vi "Get TimeStamp from NTP.vi"(8 "error in (no error)":errorcluster, 11 "Time Server\nIP Address":string="192.168.1.43") -> (0 "error out":errorcluster, 1 "Time Server\nUsed":string, 2 "Time Server\nRequested":string, 3 "Returned\nTime Stamp":timestamp format="%<%c>T")   [LabVIEW 2011]
doc: "Gets the time using the NTP protocol and sets the RT clock to that time"
uses:
  <vilib>/NI_Real-Time Target Support.lvlib
panel:
  in  "Inhibit inverse DNS":bool=TRUE
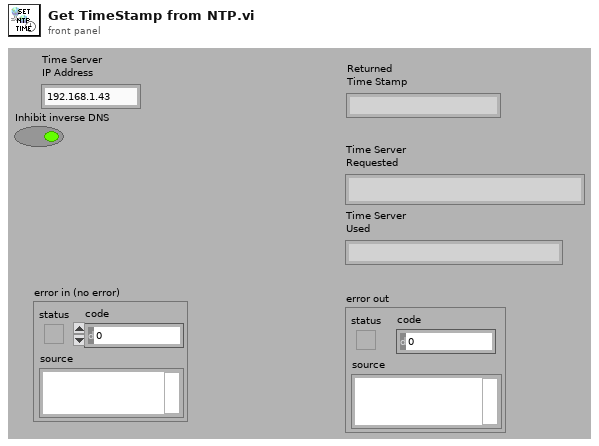
[diagram p1: front panel]
types:
  T1 = typedef "LVDateTimeRec.ctl" = cluster{"fractional second":dbl, "second":i32, "minute":i32, "hour":i32, "day of month":i32, "month":i32, "year":i32, "day of week":i32, "day of year":i32, "DST":i32}
  T2 = enum16{"set date", "set local time", "set UTC time"}
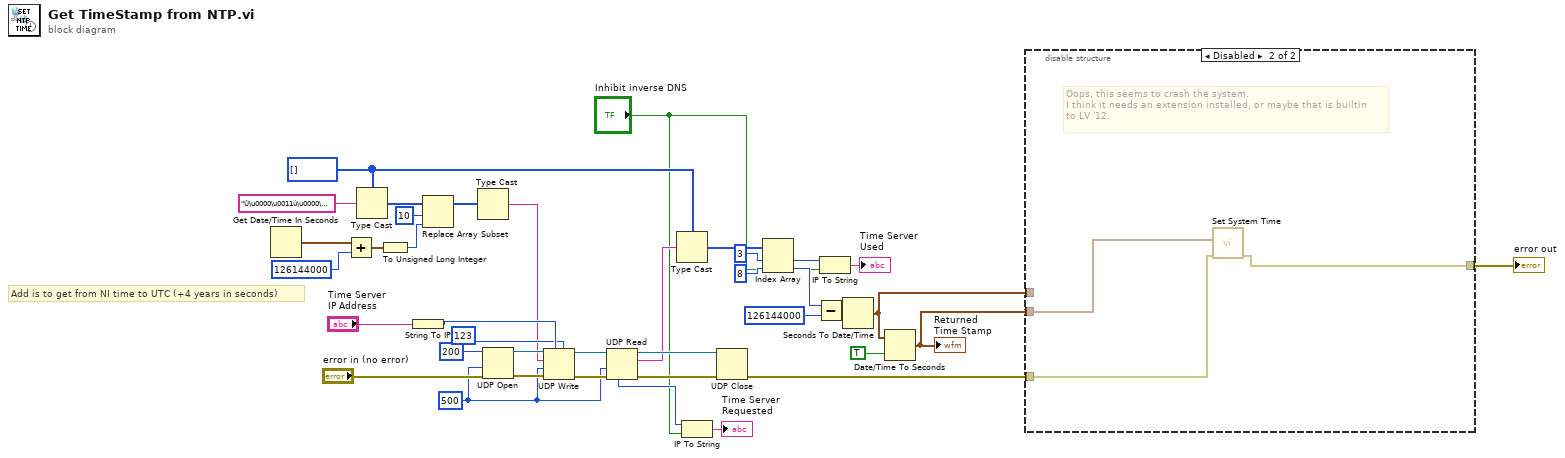
[diagram p0: block diagram]
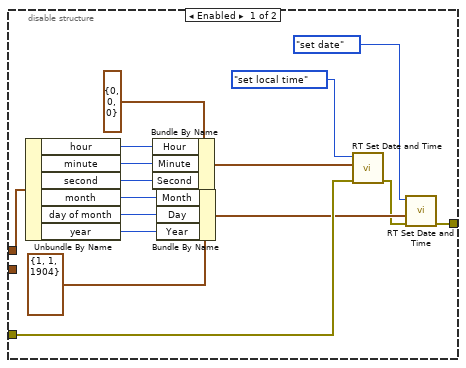
[diagram p2: hidden frame]
diagram:
  w3 = 500 ("timeout ms (25000)")
  w6 = u32[] []
  # "Add is to get from NI time to UTC (+4 years in seconds)"
  n1 = Get Date/Time In Seconds() -> (seconds since 1Jan1904=w24:timestamp)
  n2 = Add(x=w24, y=u32 126144000) -> (x+y=w19:timestamp)
  n3 = Type Cast(type=w6, x="Û\u0000\u0011ú\u0000\u0000\u0000\u0000\u0000\u0001\u0003þ\u0000\u0000\u0000\u0000Ð!ú*\u0017KÆ§\u0000\u0000\u0000\u0000\u0000\u0000\u0000\u0000\u0000\u0000\u0000\u0000\u0000\u0000\u0000\u0000Ð'l\u001a‚MÒñ€:\u0000\u0000\u0000\u0000\u0000\u0000\u0000\u0000\u0000\u0000\u0000\u0000\u0000\u0000\u0000\u0000\u0000\u0000" ("String")) -> (*(type *) &x=w22:u32[])
  n4 = To Unsigned Long Integer(number=w19) -> (unsigned 32bit integer=w13:u32)
  n5 = String To IP(1:"Time Server\nIP Address") -> (0:w36:u32)
  n6 = Replace Array Subset(array=w22, new element=w13, index=10) -> (w21:u32[])
  n7 = Type Cast(x=w21) -> (*(type *) &x=w16:string)  [unwired: 1 in]
  n8 = UDP Open(8:"error in (no error)", 9:w3, 11:u16 200 ("port")) -> (port=w37:refnum<k16>, 0:w38:errorcluster)  [unwired: 2 in, 1 out]
  n9 = UDP Write(address=w36, port or service name=u16 123 ("port"), connection ID=w37, data in=w16, 8:w38, 9:w3) -> (error out=w35:errorcluster, 3:w34:refnum<k16>)
  n10 = UDP Read(connection ID=w34, timeout ms (25000)=w3, 8:w35) -> (data out=w27:string, error out=w32:errorcluster, 3:w33:refnum<k16>, 6:w29:u32)  [unwired: 1 in, 1 out]
  n11 = Type Cast(type=w6, x=w27) -> (*(type *) &x=w26:u32[])
  n12 = IP To String(1:"Inhibit inverse DNS", 2:w29) -> (0:→"Time Server\nRequested":string)
  n13 = UDP Close(connection ID=w33, 8:w32) -> (error out=w11:errorcluster)  [unwired: 1 out]
  n14 = Index Array(array=w26, index #1=3 ("index"), index #2=8 ("index")) -> (element #1=w12:u32, element #2=w8:u32)
  n15 = Subtract(x=w8, y=u32 126144000) -> (x-y=w15:u32)
  n16 = IP To String(1:"Inhibit inverse DNS", 2:w12) -> (0:→"Time Server\nUsed":string)
  n17 = Seconds To Date/Time(time stamp (now)=w15) -> (date time rec=w5:T1)  [unwired: 1 in]
  n18 = Date/Time To Seconds(1:TRUE ("is UTC (F)"), 2:w5) -> (0:w1:timestamp)
  "Returned\nTime Stamp" <- w1
  n19 = disable-structure shown="Disabled" {
    disable-tunnel: w11 -> [w50 w58]
    disable-tunnel: [w44 w57] -> w10
    disable-tunnel: w5 -> [w43 _]
    disable-tunnel: w1 -> [_ w56]
    frame Enabled {
      n20 = Unbundle By Name(w43) -> ("hour"=w53:i32, "minute"=w52:i32, "second"=w51:i32, "month"=w48:i32, "day of month"=w47:i32, "year"=w46:i32)
      n21 = Bundle By Name(cluster=cluster{"Hour":i32, "Minute":i32, "Second":i32} {"Hour"=0, "Minute"=0, "Second"=0} ("Time"), "Hour"=w53, "Minute"=w52, "Second"=w51) -> (w54:cluster{"Hour":i32, "Minute":i32, "Second":i32})
      n22 = Bundle By Name(cluster=cluster{"Month":i32, "Day":i32, "Year":i32} {"Month"=1, "Day"=1, "Year"=1904} ("Date"), "Month"=w48, "Day"=w47, "Year"=w46) -> (w45:cluster{"Month":i32, "Day":i32, "Year":i32})
      n23 = call <vilib>:"RT Set Date and Time.vi"("error in (no error)"=w50, "Time"=w54, "mode"=T2."set local time") -> ("error out"=w41:errorcluster)  [unwired: 8 in]
      n24 = call <vilib>:"RT Set Date and Time.vi"("error in (no error)"=w41, "Date"=w45, "mode"=T2."set date") -> ("error out"=w44:errorcluster)  [unwired: 8 in]
    }
    frame Disabled {
      # "Oops, this seems to crash the system.\nI think it needs an extension installed, or maybe that is builtin\nto LV '12."
      n25 = call "Set System Time.vi"("error in (no error)"=w58, "Time:Current time"=w56) -> ("error out"=w57:errorcluster)  [unwired: 6 in, 3 out]
    }
  }
  "error out" <- w10
